vi "GPack Exists.vi"(10 "Folder":path) -> (2 "Has GPack":bool)   [LabVIEW 2020, in "GPack.lvlib" / "PackageAbstract.lvclass"]
uses:
  PackageAbstract.lvclass
  GPack File/GPack File.lvclass
  PackageAbstract.lvclass/PackageAbstract.ctl
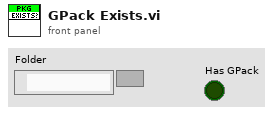
[diagram p1: front panel]
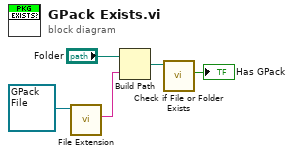
[diagram p0: block diagram]
diagram:
  n1 = call-dynamic "File Extension.vi"("GPack File in"=refnum<class "GPack File.lvclass"> refnum ("GPack.lvlib:GPack File.lvclass")) -> ("File Extension"=w3:string)  [unwired: 9 in, 1 out]
  n2 = Build Path(base path="Folder", name or relative path=w3) -> (appended path=w2:path)
  n3 = call <vilib>:"Check if File or Folder Exists.vi"("path"=w2) -> ("file or folder exists?"=→"Has GPack":bool)  [unwired: 8 in, 2 out]
